vi "dfd_Specific TF Validation.vi"(8 "error in (no error)":errorcluster, 9 "type":T1, 10 "denominator":dbl[](array[numeric]) format="%.2f", 11 "numerator":dbl[](array[numeric]) format="%.2f") -> (0 "error out":errorcluster, 2 "dup denominator":dbl[](array[numeric]) format="%.2f", 3 "dup numerator":dbl[](array[numeric]) format="%.2f")   [LabVIEW 2017, in "NI_DigFilterLicensed.lvlib"]
uses:
  <vilib>/addons/Digital Filter Design/NI_DigFilterLicensed.lvlib
  <vilib>/addons/Digital Filter Design/_Objects.llb/DFD Filter Structure Type Selector.ctl
  <vilib>/addons/Digital Filter Design/_Misc.llb/dfd_Error Handlers (Single).vi
  <vilib>/addons/Digital Filter Design/_Misc.llb/dfd_X Equal Y (Array).vi
  <vilib>/Analysis/polynomials.llb/Polynomial Roots (DBL).vi
  <vilib>/Analysis/NI_AALPro.lvlib
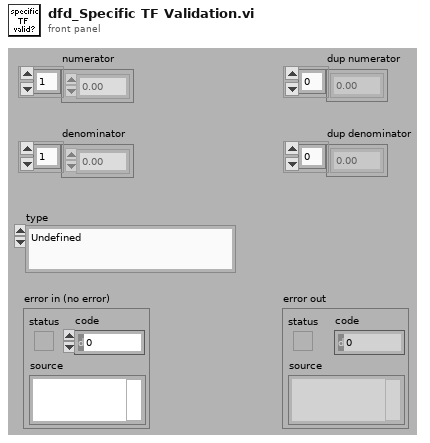
[diagram p1: front panel]
types:
  T1 = typedef "NI_DigFilterLicensed.lvlib/DFD Filter Structure Type Selector.ctl" = enum16{"Undefined", "FIR Direct Form", "FIR Direct Form Transposed", "FIR Symmetric", "FIR Antisymmetric", "IIR Direct Form I", "IIR Direct Form I Transposed", "IIR Direct Form II", "IIR Direct Form II Transposed", "IIR Cascaded Second Order Sections Form I", "IIR Cascaded Second Order Sections Form I Transposed", "IIR Cascaded Second Order Sections Form II", "IIR Cascaded Second Order Sections Form II Transposed", "Lattice Allpass (basic sections)", "Lattice Allpass (one multiplier sections)", "Lattice Allpass (normalized sections)", "Lattice AR (basic sections)", "Lattice AR (one multiplier sections)", "Lattice AR (normalized sections)", "Lattice MA (minimum phase)", "Lattice MA (maximum phase)", "Lattice ARMA (basic sections)", "Lattice ARMA (one multiplier sections)", "Lattice ARMA (normalized sections)"}
  T2 = typedef "NI_DigFilterLicensed.lvlib/DFD Filter Structure Id.ctl" = enum16{"Undefined", "FIR", "IIR Direct", "IIR SOS", "IIR Allpass", "IIR AR", "IIR ARMA"}
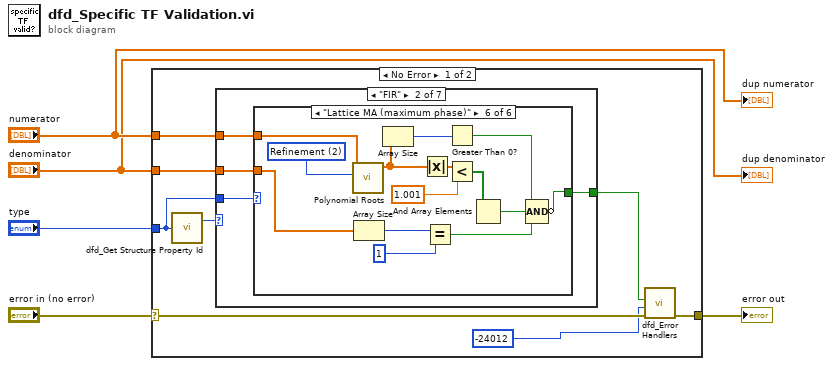
[diagram p0: block diagram]
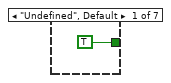
[diagram p2: hidden frame]
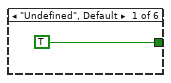
[diagram p3: hidden frame]
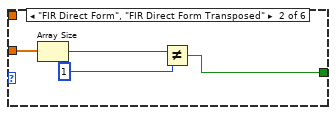
[diagram p4: hidden frame]
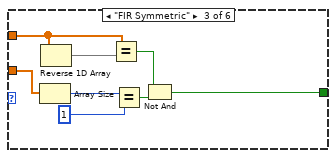
[diagram p5: hidden frame]
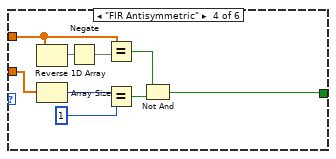
[diagram p6: hidden frame]
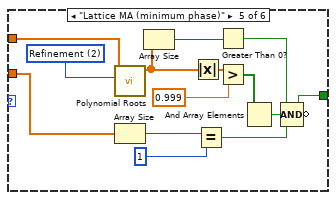
[diagram p7: hidden frame]
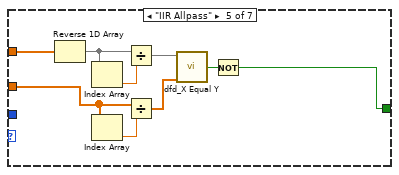
[diagram p10: hidden frame]
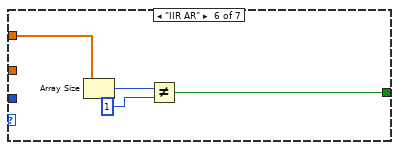
[diagram p11: hidden frame]
diagram:
  n1 = case shown="No Error" "error in (no error)" {
    selector: "error in (no error)" -> [w9 w82]
    tunnel: "type" -> [w10 _]
    tunnel: [w8 w82] -> w3
    tunnel: "numerator" -> [w12 _]
    tunnel: "denominator" -> [w11 _]
    frame No Error {
      n2 = call <vilib>:"dfd_Get Structure Property Id.vi"("structure type"=w10) -> ("filter structure id"=w13:T2)  [unwired: 1 out]
      n3 = case shown="\"FIR\"" w13 {
        tunnel: w12 -> [_ w17 _ _ w74 w79 _]
        tunnel: w11 -> [_ w16 _ _ w73 _ _]
        tunnel: w10 -> [_ w18 _ _ _ _ _]
        tunnel: [TRUE w15 _ _ w70 w78 _] -> w7
        frame "Undefined", Default {
        }
        frame "FIR" {
          n4 = case shown="\"Lattice MA (maximum phase)\"" w18 {
            tunnel: w17 -> [_ _ w30 w38 w43 w57]
            tunnel: w16 -> [_ w23 w29 w37 w49 w63]
            tunnel: [TRUE w20 w24 w32 w42 w56] -> w15
            frame "Undefined", Default {
            }
            frame "FIR Direct Form", "FIR Direct Form Transposed" {
              n5 = Array Size(array=w23) -> (size(s)=w22:i32)
              n6 = Not Equal?(x=w22, y=1) -> (x != y?=w20:bool)
            }
            frame "FIR Symmetric" {
              n7 = Array Size(array=w29) -> (size(s)=w28:i32)
              n8 = Reverse 1D Array(array=w30) -> (reversed array=w31:dbl[])
              n9 = Equal?(x=w30, y=w31) -> (x = y?=w25:bool)
              n10 = Equal?(x=w28, y=1) -> (x = y?=w26:bool)
              n11 = Not And(1:w26, 2:w25) -> (0:w24:bool)
            }
            frame "FIR Antisymmetric" {
              n12 = Reverse 1D Array(array=w38) -> (reversed array=w40:dbl[])
              n13 = Array Size(array=w37) -> (size(s)=w36:i32)
              n14 = Negate(x=w40) -> (-x=w39:dbl[])
              n15 = Equal?(x=w38, y=w39) -> (x = y?=w33:bool)
              n16 = Equal?(x=w36, y=1) -> (x = y?=w34:bool)
              n17 = Not And(1:w34, 2:w33) -> (0:w32:bool)
            }
            frame "Lattice MA (minimum phase)" {
              w41 = u16 2 items=["General", "Simple Classification", "Refinement", "Advanced Refinement"] ("option")
              n18 = call-poly <vilib>:"Polynomial Roots.vi"("option"=w41, "P(x)"=w43) -> ("Roots"=w50:cdb[])  [unwired: 1 in, 8 out]
              n19 = Array Size(array=w49) -> (size(s)=w48:i32)
              n20 = Array Size(array=w50) -> (size(s)=w51:i32)
              n21 = Absolute Value(x=w50) -> (abs(x)=w54:dbl[])
              n22 = Equal?(x=w48, y=1) -> (x = y?=w44:bool)
              n23 = Greater Than 0?(x=w51) -> (x > 0?=w46:bool)
              n24 = Greater?(x=w54, y=0.999) -> (0:w52:bool[])
              n25 = And Array Elements(Boolean array=w52) -> (logical AND=w45:bool)
              n26 = Compound Arithmetic op=AND(w46, w45, w44) -> (invert w42:bool)
            }
            frame "Lattice MA (maximum phase)" {
              w55 = u16 2 items=["General", "Simple Classification", "Refinement", "Advanced Refinement"] ("option")
              n27 = call-poly <vilib>:"Polynomial Roots.vi"("option"=w55, "P(x)"=w57) -> ("Roots"=w64:cdb[])  [unwired: 1 in, 8 out]
              n28 = Array Size(array=w63) -> (size(s)=w62:i32)
              n29 = Array Size(array=w64) -> (size(s)=w65:i32)
              n30 = Absolute Value(x=w64) -> (abs(x)=w68:dbl[])
              n31 = Equal?(x=w62, y=1) -> (x = y?=w58:bool)
              n32 = Greater Than 0?(x=w65) -> (x > 0?=w60:bool)
              n33 = Less?(x=w68, y=1.001) -> (x < y?=w66:bool[])
              n34 = And Array Elements(Boolean array=w66) -> (logical AND=w59:bool)
              n35 = Compound Arithmetic op=AND(w60, w59, w58) -> (invert w56:bool)
            }
          }
        }
        frame "IIR Direct" {
        }
        frame "IIR SOS" {
        }
        frame "IIR Allpass" {
          n36 = Reverse 1D Array(array=w74) -> (reversed array=w77:dbl[])
          n37 = Index Array(array=w77) -> (element=w76:dbl)  [unwired: 1 in]
          n38 = Index Array(array=w73) -> (element=w75:dbl)  [unwired: 1 in]
          n39 = Divide(x=w77, y=w76) -> (x/y=w72:dbl[])
          n40 = Divide(x=w73, y=w75) -> (x/y=w71:dbl[])
          n41 = call-poly <vilib>:"dfd_X Equal Y.vi"("x"=w72, "y"=w71) -> ("x = y?"=w69:bool)  [unwired: 1 in, 4 out]
          n42 = Not(x=w69) -> (.not. x?=w70:bool)
        }
        frame "IIR AR" {
          n43 = Array Size(array=w79) -> (size(s)=w81:i32)
          n44 = Not Equal?(x=w81, y=1) -> (x != y?=w78:bool)
        }
        frame "IIR ARMA" {
        }
      }
      n45 = call-poly <vilib>:"dfd_Error Handlers.vi"("error in (no error)"=w9, "error code"=-24012 ("ERR_INCOMPATIBLE_STRUT"), "condition failed?"=w7) -> ("error out"=w8:errorcluster)  [unwired: 8 out]
    }
    frame Error {
    }
  }
  "error out" <- w3
  "dup numerator" <- "numerator"
  "dup denominator" <- "denominator"
